vi "AlliGator Check HDF5 Image Size v2.vi"(9 "Image Binning Options":T1={"Use Image Binning"=FALSE, "X Bin"=1, "Y Bin"=1} {"Y Bin" min=1; "X Bin" min=1}, 10 "Image ROI Information":T2, 11 "FLI Parameters in":T3) -> (3 "FLI Parameters out":T3)   [LabVIEW 2021, in "AlliGator HDF5.lvlib"]
doc: "Determines the gate image dimension (X, Y) from the provided file information."
uses:
  AlliGator HDF5.lvlib
  Phasor/Phasor Fluorescence Lifetime Parameters v3.ctl
  SwissSPAD/SwissSPAD Live_Image ROI Information.ctl
  AlliGator Image Binning Options.ctl
  SwissSPAD/SwissSPAD Live.lvlib
  AlliGator Source Image.lvlib
  Phasor/Phasor.lvlib
panel:
  # "see the AlliGator License on the block diagram (Ctrl+E or Window:Show Block Diagram)"
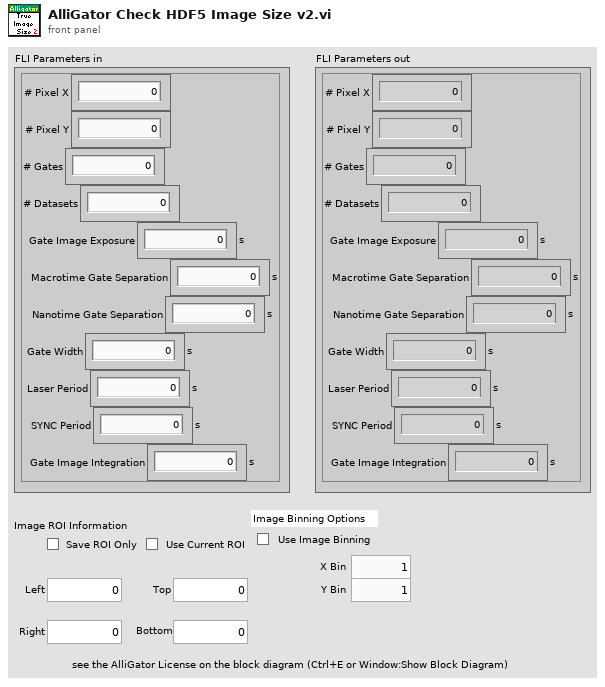
[diagram p1: front panel]
types:
  T1 = typedef "AlliGator Source Image.lvlib/AlliGator Image Binning Options.ctl" = cluster{"Use Image Binning":bool, "X Bin":i32, "Y Bin":i32}
  T2 = typedef "SwissSPAD Live.lvlib/SwissSPAD Live_Image ROI Information.ctl" = cluster{"Save ROI Only":bool, "Left":u16, "Top":u16, "Right":u16, "Bottom":u16, "Use Current ROI":bool}
  T3 = typedef "Phasor.lvlib/Phasor Fluorescence Lifetime Parameters v3.ctl" = cluster{"# Pixel X":i32, "# Pixel Y":i32, "# Gates":i32, "# Datasets":i32, "Gate Image Exposure":dbl[unit], "Macrotime Gate Separation":dbl[unit], "Nanotime Gate Separation":dbl[unit], "Gate Width":dbl[unit], "Laser Period":dbl[unit], "SYNC Period":dbl[unit], "Gate Image Integration":dbl[unit]}
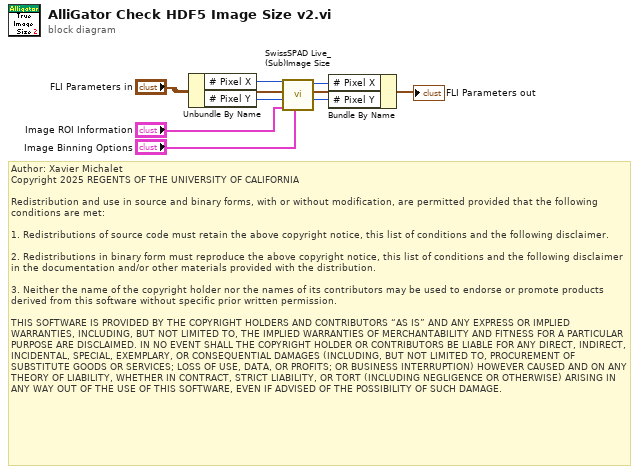
[diagram p0: block diagram]
diagram:
  # "Author: Xavier Michalet\nCopyright 2025 REGENTS OF THE UNIVERSITY OF CALIFORNIA\n\nRedistribution and use in source and binary forms, with or without modification, are permitted provided that the following conditions are met:\n\n1. Redistributions of source code must retain the above copyright notice, this list of conditions and the following disclaimer.\n\n2. Redistributions in binary form must reproduce the above copyright notice, this list of conditions and the following disclaimer in the documentation and/or other materials provided with the distribution.\n\n3. Neither the name of the copyright holder nor the names of its contributors may be used to endorse or promote products derived from this software without specific prior written permission.\n\nTHIS SOFTWARE IS PROVIDED BY THE COPYRIGHT HOLDERS AND CONTRIBUTORS “AS IS” AND ANY EXPRESS OR IMPLIED WARRANTIES, INCLUDING, BUT NOT LIMITED TO, THE IMPLIED WARRANTIES OF MERCHANTABILITY AND FITNESS FOR A PARTICULAR PURPOSE ARE DISCLAIMED. IN NO EVENT SHALL THE COPYRIGHT HOLDER OR CONTRIBUTORS BE LIABLE FOR ANY DIRECT, INDIRECT, INCIDENTAL, SPECIAL, EXEMPLARY, OR CONSEQUENTIAL DAMAGES (INCLUDING, BUT NOT LIMITED TO, PROCUREMENT OF SUBSTITUTE GOODS OR SERVICES; LOSS OF USE, DATA, OR PROFITS; OR BUSINESS INTERRUPTION) HOWEVER CAUSED AND ON ANY THEORY OF LIABILITY, WHETHER IN CONTRACT, STRICT LIABILITY, OR TORT (INCLUDING NEGLIGENCE OR OTHERWISE) ARISING IN ANY WAY OUT OF THE USE OF THIS SOFTWARE, EVEN IF ADVISED OF THE POSSIBILITY OF SUCH DAMAGE."
  n1 = Unbundle By Name("FLI Parameters in") -> ("# Pixel X"=w8:i32, "# Pixel Y"=w7:i32)
  n2 = call "SwissSPAD Live_(Sub)Image Size.vi"("Image Binning Options"="Image Binning Options", "Image Information"="Image ROI Information", "# Pixel Y in"=w7, "# Pixel X in"=w8) -> ("# Pixel Y out"=w3:i32, "# Pixel X out"=w4:i32)  [unwired: 6 in]
  n3 = Bundle By Name(cluster="FLI Parameters in", "# Pixel X"=w4, "# Pixel Y"=w3) -> (→"FLI Parameters out":T3)
